vi "kepcoScanStandAloneHostTest.vi"() -> ()   [LabVIEW 2014]
uses:
  <vilib>/FPGAPlugInAG/PXI-7852R/niLvFpga_Open_PXI-7852R.vi
  <vilib>/rvi/interface/common/dynamic/niFpgaDynamicAddResources.vi
  <vilib>/Utility/error.llb/Error Cluster From Error Code.vi
  <vilib>/rvi/errors/niLvFpgaAdjustHostInterfaceError.vi
  <vilib>/FPGAPlugInAG/Dynamic/niLvFpga_Close_Dynamic.vi
  <vilib>/rvi/interface/nirviOpenFPGA/nirviOpenFPGA.xnode
  FPGA Bitfiles/TiTaProj_DAF_kepcoScanStandAlone.lvbitx
  <vilib>/rvi/interface/nirviReadWriteControl/nirviReadWriteControl.xnode
  <vilib>/rvi/interface/nirviMethod/nirviMethod.xnode
  <vilib>/rvi/interface/nirviCloseFPGA/nirviCloseFPGA.xnode
  NiFpgaLv.dll
  <vilib>/rvi/interface/Simulation/niFpgaSimulationCallBeginRW.vi
  <vilib>/FPGAPlugInAG/Dynamic/niLvFpga_WriteFifo_Dynamic.vi
  <vilib>/rvi/errors/niLvFpgaMergeErrorWithErrorCode.vi
panel:
  in  "SetValuesforNextScan":bool=TRUE
  in  "invertInOddnOfTrack":bool
  out "i outer":i32
  in  "waitAfterReset(25nsTicks)":u16
  in  "Go":bool
  in  "abort":bool
  out "timeoutDAC":bool
  in  "Data":i32[](array[numeric])=[65536, 1048576, 4, 3, 32768, 1572864, 5, 2, 16384, 1310720, 6, 2] format="%024b"
  in  "nOfScanRegions":i32=1
  in  "waitForKepco(25nsTicks)":u16=1
  in  "waitForDmm(ms)":dbl=1.0
  # "Each  scan region consists of: [step, start, nOfSteps, nOfTracks]"
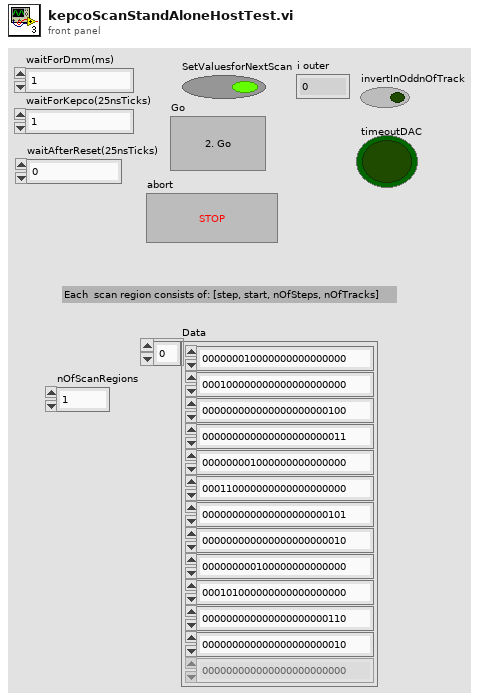
[diagram p1: front panel]
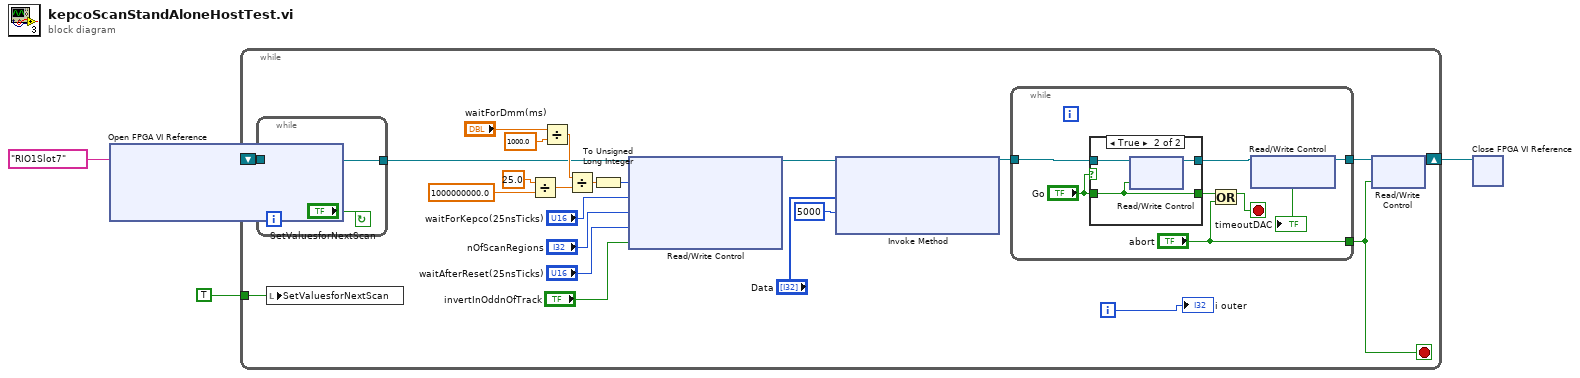
[diagram p0: block diagram]
diagram:
  n1 = xnode ("Open FPGA VI Reference")("resource name"=tag "RIO1Slot7") -> ("FPGA VI Reference Out"=w4:refnum<k20>)  [unwired: 1 in, 1 out]
  n2 = while {
    shift-right: [w10] -> w3
    shift-left: w4 -> [w7]
    tunnel: TRUE ("SetValuesforNextScan") -> [w5]
    i -> [w9]
    stop <- w8 stop-if-true
    n3 = while {
      tunnel: w7 -> [w29]
      tunnel: [w29] -> w6
      stop <- "SetValuesforNextScan" continue-if-true
    }
    n4 = local write "SetValuesforNextScan"(w5) -> ()
    n5 = Divide(x=25.0 ("y"), y=1000000000.0) -> (x/y=w23:dbl)
    n6 = Divide(x="waitForDmm(ms)", y=1000.0) -> (x/y=w25:dbl)
    n7 = Divide(x=w25, y=w23) -> (x/y=w21:dbl)
    n8 = To Unsigned Long Integer(number=w21) -> (unsigned 32bit integer=w16:u32)
    n9 = xnode "Read/Write Control"("FPGA VI Reference In"=w6, "waitForDmm(25nsTicks)"=w16, "waitForKepco(25nsTicks)"="waitForKepco(25nsTicks)", "nOfScanRegions"="nOfScanRegions", "waitAfterReset(25nsTicks)"="waitAfterReset(25nsTicks)", "invertInOddnOfTrack"="invertInOddnOfTrack") -> ("FPGA VI Reference Out"=w15:refnum<k20>)  [unwired: 1 in, 1 out]
    n10 = xnode "Invoke Method"("FPGA VI Reference In"=w15, "Data"="Data", "Timeout (ms)"=5000) -> ("FPGA VI Reference Out"=w12:refnum<k20>)  [unwired: 1 in, 2 out]
    n11 = while {
      tunnel: w12 -> [w37]
      tunnel: [w34] -> w19
      tunnel: ["abort"] -> w8
      stop <- w31 stop-if-true
      n12 = case shown="True" "Go" {
        tunnel: w37 -> [w39 w42]
        tunnel: [w39 w41] -> w36
        tunnel: "Go" -> [w38 w40]
        tunnel: [w38 w40] -> w32
        frame False {
        }
        frame True {
          n13 = xnode "Read/Write Control"("FPGA VI Reference In"=w42, "Go"=w40) -> ("FPGA VI Reference Out"=w41:refnum<k20>)  [unwired: 1 in, 1 out]
        }
      }
      n14 = Or(x=w32, y="abort") -> (x .or. y?=w31:bool)
      n15 = xnode "Read/Write Control"("FPGA VI Reference In"=w36) -> ("FPGA VI Reference Out"=w34:refnum<k20>, "timeoutDAC"=→"timeoutDAC":bool)  [unwired: 1 in, 1 out]
    }
    n16 = xnode "Read/Write Control"("FPGA VI Reference In"=w19, "abort"=w8) -> ("FPGA VI Reference Out"=w10:refnum<k20>)  [unwired: 1 in, 1 out]
    "i outer" <- w9
  }
  n17 = xnode "Close FPGA VI Reference"("FPGA VI Reference In"=w3) -> ()  [unwired: 1 in, 1 out]
